vi "No Timeout.vi"(7 "Ignore Control":T1, 8 "error in (no error)":errorcluster) -> (0 "error out":errorcluster, 4 "Timeout":bool, 6 "Error Code Out":i32)   [LabVIEW 2011]
uses:
  Ignore Control Cluster.ctl
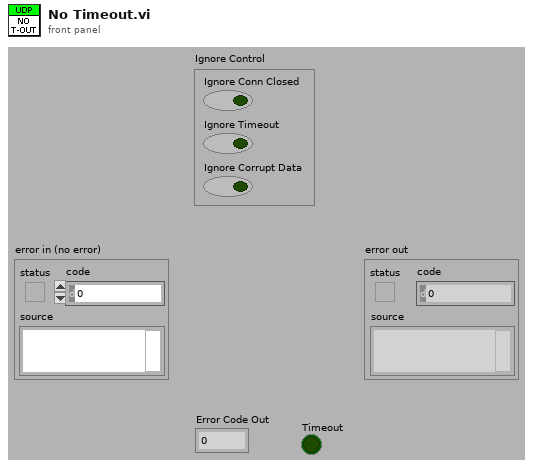
[diagram p1: front panel]
types:
  T1 = typedef "Ignore Control Cluster.ctl" = cluster{"Ignore Conn Closed":bool, "Ignore Timeout":bool, "Ignore Corrupt Data":bool}
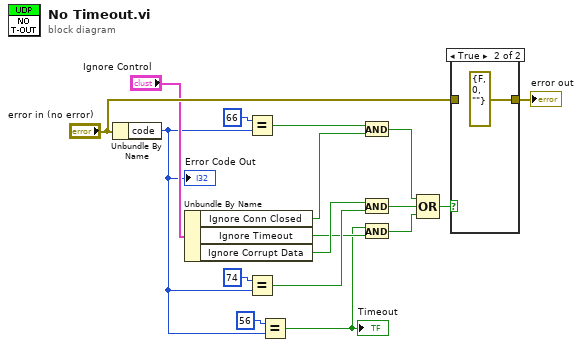
[diagram p0: block diagram]
diagram:
  n1 = Unbundle By Name("error in (no error)") -> ("code"=w10:i32)
  "Error Code Out" <- w10
  n2 = Unbundle By Name("Ignore Control") -> ("Ignore Conn Closed"=w9:bool, "Ignore Timeout"=w5:bool, "Ignore Corrupt Data"=w8:bool)
  n3 = Equal?(x=66, y=w10) -> (x = y?=w6:bool)
  n4 = Equal?(x=74, y=w10) -> (x = y?=w7:bool)
  n5 = Equal?(x=56, y=w10) -> (x = y?=w1:bool)
  "Timeout" <- w1
  n6 = And(x=w6, y=w9) -> (x .and. y?=w2:bool)
  n7 = And(x=w8, y=w7) -> (x .and. y?=w4:bool)
  n8 = And(x=w1, y=w5) -> (x .and. y?=w3:bool)
  n9 = Compound Arithmetic op=OR(w2, w4, w3) -> (w15:bool)
  n10 = case shown="True" w15 {
    tunnel: "error in (no error)" -> [w18 _]
    tunnel: [w18 errorcluster {"status"=FALSE, "code"=0, "source"=""} ("error out")] -> w13
    frame False {
    }
    frame True {
    }
  }
  "error out" <- w13
